vi "sub vi - temperature delay v1.vi"() -> ()   [LabVIEW 2013]
uses:
  <vilib>/Platform/TimedLoop/XDataNode/timing_clust.ctl
  <vilib>/Platform/TimedLoop/XDataNode/nitl_modes.ctl
  <vilib>/Platform/TimedLoop/XDataNode/wakeup.ctl
  <vilib>/platform/TimedLoop/XDataNode/XDataNode.xnode
  <vilib>/Platform/TimedLoop/XDataNode/XDNodeRunTimeDep.lvlib
panel:
  out "cycle":bool
  out "count":dbl
  out "temp":dbl
  in  "Numeric Control":dbl
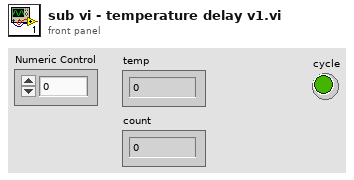
[diagram p1: front panel]
types:
  T1 = typedef "XDNodeRunTimeDep.lvlib/timing_clust.ctl" = cluster{"Expected End [f-1]":u64, "Actual End [f-1]":u64, "Finished Late? [f-1]":bool, "Expected End [i-1]":u64, "Actual End [i-1]":u64, "Finished Late? [i-1]":bool, "Expected Start [i]":u64, "Actual Start [i]":u64, "Expected Start [f]":u64, "Actual Start [f]":u64, "Source Name":string, "Structure Name":string, "Period":i64, "Deadline":i64, "Offset":i64, "Start":i64, "Priority":i32, "Timeout":i32, "Mode":T2, "Wakeup Reason":T3, "Error":errorcluster, "Source Type":string, "Secondary Source Type":string, "Global End Time":u64, "Global Start Time":u64, "Frame Duration":u64, "Iteration Duration":u64, "Assigned CPU":i32, "I/O Scan Engine Mode":u32}
  T2 = typedef "XDNodeRunTimeDep.lvlib/nitl_modes.ctl" = enum32{"No Change", "Process missed periods, maintain original phase", "Discard missed periods, maintain original phase", "Process missed periods, ignore original phase", "Discard missed periods, ignore original phase"}
  T3 = typedef "XDNodeRunTimeDep.lvlib/wakeup.ctl" = enum32{"Normal", "Aborted", "Asynchronous wakeup", "Timing source error", "Timed loop error", "Timeout"}
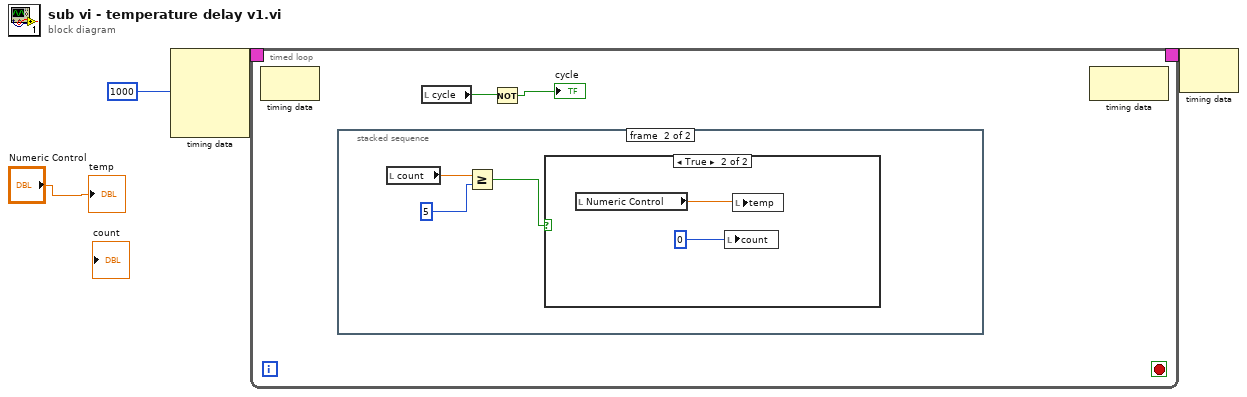
[diagram p0: block diagram]
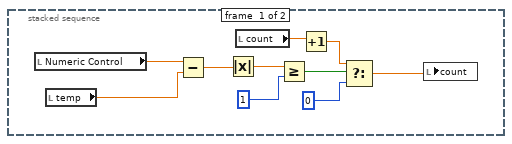
[diagram p2: hidden frame]
diagram:
  n1 = node-c288(1000) -> (w4:T1)  [unwired: 3 in]
  n2 = timed-loop {
    timing: w4 -> [_]
    timing-out: [_] -> w3
    stop <- _ stop-if-true
    n3 = node-c288() -> ()  [unwired: 1 in, 1 out]
    n4 = stacked-sequence {
      frame #0 {
        n5 = local read "Numeric Control"() -> (w16:dbl)
        n6 = local read "temp"() -> (w15:dbl)
        n7 = Subtract(x=w16, y=w15) -> (x-y=w14:dbl)
        n8 = Absolute Value(x=w14) -> (abs(x)=w13:dbl)
        n9 = local read "count"() -> (w10:dbl)
        n10 = Greater Or Equal?(x=w13, y=1) -> (x >= y?=w11:bool)
        n11 = Increment(x=w10) -> (x+1=w9:dbl)
        n12 = Select(t=w9, s=w11, f=0) -> (s? t:f=w8:dbl)
        n13 = local write "count"(w8) -> ()
      }
      frame #1 {
        n14 = local read "count"() -> (w19:dbl)
        n15 = Greater Or Equal?(x=w19, y=5) -> (x >= y?=w17:bool)
        n16 = case shown="True" w17 {
          frame False {
          }
          frame True {
            n17 = local read "Numeric Control"() -> (w21:dbl)
            n18 = local write "count"(0) -> ()
            n19 = local write "temp"(w21) -> ()
          }
        }
      }
    }
    n20 = local read "cycle"() -> (w6:bool)
    n21 = Not(x=w6) -> (.not. x?=→"cycle":bool)
    n22 = node-c288() -> ()  [unwired: 1 in, 1 out]
  }
  n23 = node-c288(w3) -> ()  [unwired: 1 out]
  "temp" <- "Numeric Control"
